vi "Math.Check if in Tolerance.vi"(6 "Include Limits":bool, 9 "Limit %":dbl=1.0, 10 "Actual":dbl, 11 "Target":dbl) -> (0 "Error %":dbl=1.0, 1 "Difference(Act-Stpt)":dbl, 2 "Greater than Target":bool, 3 "In Tolerance":bool)   [LabVIEW 2024, in "EQMF.lvlib" / "Math Utils.lvlib"]
uses:
  Math Utils.lvlib
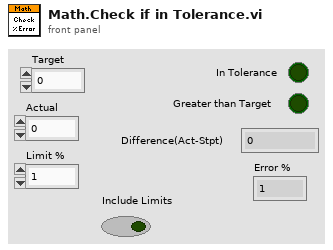
[diagram p1: front panel]
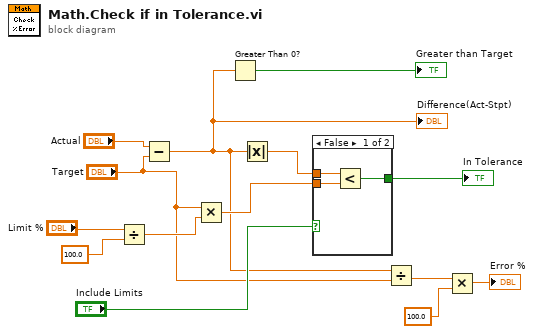
[diagram p0: block diagram]
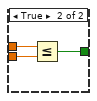
[diagram p2: hidden frame]
diagram:
  n1 = Divide(x="Limit %", y=100.0) -> (x/y=w13:dbl)
  n2 = Subtract(x="Actual", y="Target") -> (x-y=w1:dbl)
  "Difference(Act-Stpt)" <- w1
  n3 = Multiply(x="Target", y=w13) -> (x*y=w9:dbl)
  n4 = Greater Than 0?(x=w1) -> (x > 0?=→"Greater than Target":bool)
  n5 = Absolute Value(x=w1) -> (abs(x)=w3:dbl)
  n6 = case shown="False" "Include Limits" {
    tunnel: w3 -> [w17 w19]
    tunnel: w9 -> [w16 w20]
    tunnel: [w15 w18] -> w8
    frame False {
      n7 = Less?(x=w17, y=w16) -> (x < y?=w15:bool)
    }
    frame True {
      n8 = Less Or Equal?(x=w19, y=w20) -> (x <= y?=w18:bool)
    }
  }
  "In Tolerance" <- w8
  n9 = Divide(x=w1, y="Target") -> (x/y=w4:dbl)
  n10 = Multiply(x=w4, y=100.0) -> (x*y=→"Error %":dbl)
